vi "Print Test Report By Month_ABB.vi"(7 "Y Scale.Range:Maximum":dbl, 8 "To":timestamp format="%<%m/%Y>T", 9 "From":timestamp format="%<%m/%Y>T", 10 "List":string[][](array[string]), 11 "XY Graph":cluster{u64[], i32[]}(graph)) -> ()   [LabVIEW 2017]
panel:
  in  "Motors Tested":i32(listbox)
  # "Motors Tested"
  # "Motors Tested"
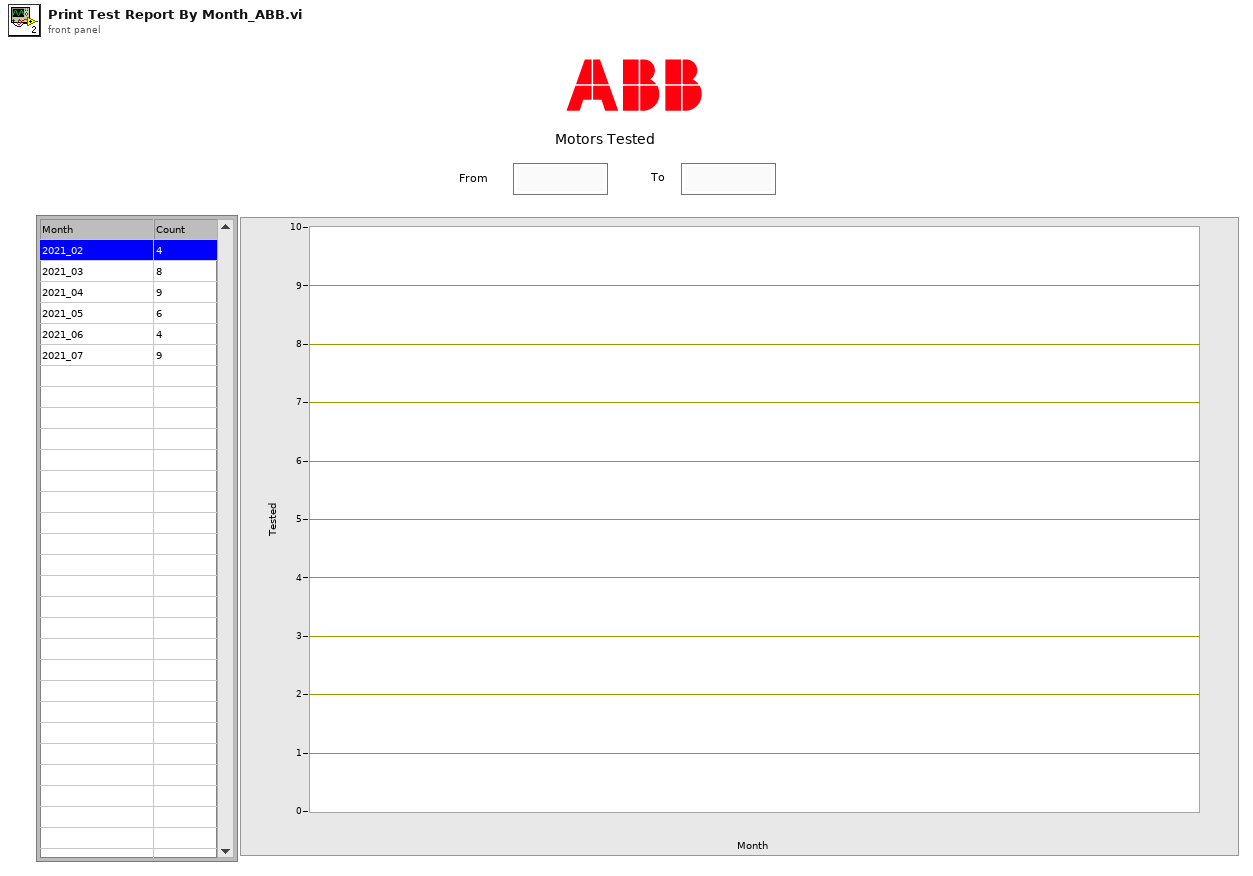
[diagram p1: front panel]
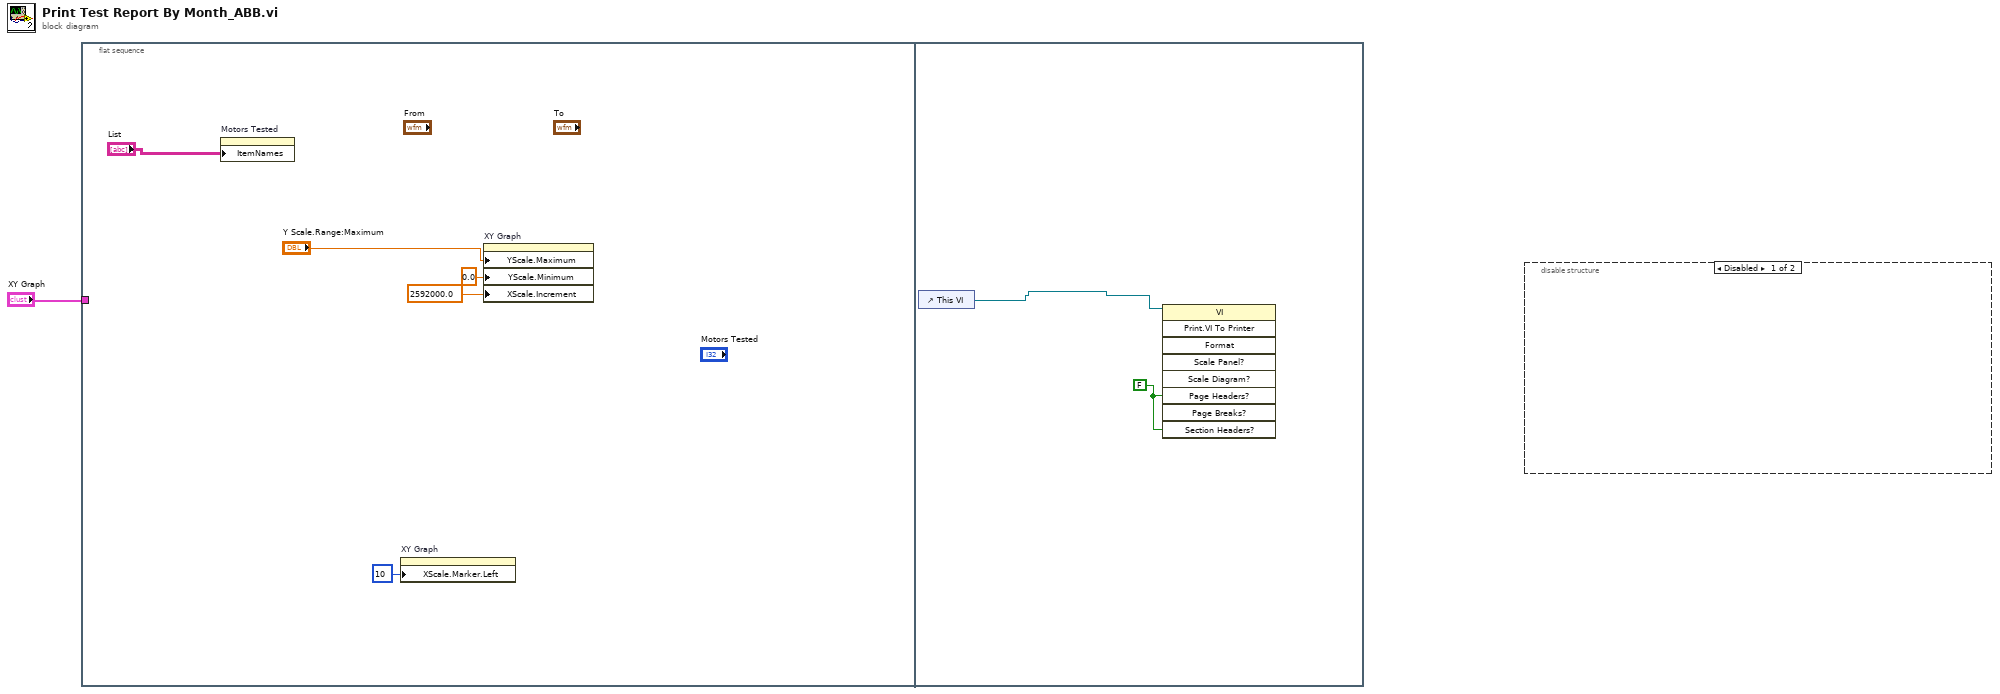
[diagram p0: block diagram]
diagram:
  n1 = flat-sequence {
    tunnel: "XY Graph" -> [_]
    frame #0 {
      n2 = property on="Motors Tested" class="MCListbox (strict)"("ItemNames"="List") -> ()  [unwired: 2 in, 2 out]
      n3 = property on="XY Graph" class="XYGraph (strict)"("XScale.Marker.Left"=10 ("X Scale.Marker.Position:Left")) -> ()  [unwired: 2 in, 2 out]
      n4 = property on="XY Graph" class="XYGraph (strict)"("YScale.Maximum"="Y Scale.Range:Maximum", "YScale.Minimum"=0.0 ("Y Scale.Range:Minimum"), "XScale.Increment"=2592000.0 ("X Scale.Range:Increment")) -> ()  [unwired: 2 in, 2 out]
    }
    frame #1 {
      w7 = FALSE ("Page Headers?")
      n5 = control-ref of="This VI"() -> (w8:refnum<vi>)
      n6 = invoke class="VI" method="Print.VI To Printer"(reference=w8, "Page Headers?"=w7, "Section Headers?"=w7) -> ()  [unwired: 6 in, 9 out]
    }
  }
  n7 = disable-structure shown="Disabled" {
    frame Disabled {
    }
    frame Enabled {
    }
  }
